vi "Initialize Attributes.vi"(8 "error in (no error)":errorcluster, 10 "Attribute Data":variant, 11 "CS++Fgen in":refnum<class "CS++Fgen.lvclass">) -> (0 "error out":errorcluster, 2 "Found?":bool, 3 "CS++Fgen out":refnum<class "CS++Fgen.lvclass">)   [LabVIEW 2016, in "CS++Fgen.lvlib" / "CS++Fgen.lvclass"]
doc: "Initialize object attribute.\n\nUnique resources should be allocated elsewhere!"
uses:
  CS++Fgen.lvclass
  C:/User/Brand/LVP/CSPP-Dev/Packages/CSPP_Core/Actors/CS++BaseActor/CS++BaseActor.lvclass
  PV-Enum.ctl
  PV-Enum-n.ctl
  CSPP_Core/Classes/CS++ProcessVariables/ProcessVariable/PV.lvclass
  CSPP_Core/Actors/CS++BaseActor/CS++BaseActor.lvclass/CS++BaseActor.ctl
  CSPP_Core/Classes/CS++ProcessVariables/ProcessVariable/PV.lvclass/PV.ctl
  CS++Fgen.lvclass/CS++Fgen.ctl
  CSPP_Core/Classes/CS++ProcessVariables/ProcessVariable/Write PV URL.vi
  CSPP_Core/Classes/CS++ProcessVariables/ProcessVariable/Write Type Descriptor.vi
  <vilib>/Utility/error.llb/Error Cluster From Error Code.vi
  CSPP_Core/Actors/CS++DeviceActor/CS++DeviceActor.lvclass
  CSPP_Core/Classes/CS++BaseClasses/Factory/CS++Factory.lvclass
  CSPP_Core/Actors/CS++BaseActor/CS++BaseActor.lvclass
  CSPP_Core/Libraries/Utilities/CS++Utilities.lvlib
  CSPP_Core/Classes/CS++ProcessVariables/CS++ProcessVariables.lvlib
panel:
  in  "PV-Enum-n":T1
  in  "PV-Enum":T2
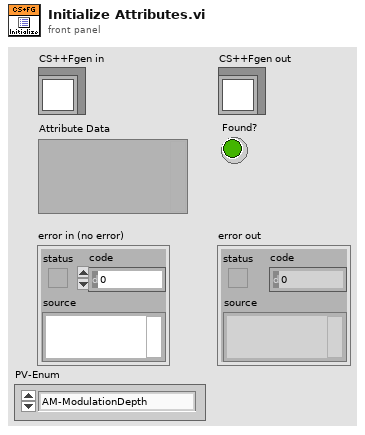
[diagram p1: front panel]
types:
  T1 = typedef "CS++Fgen.lvlib/CS++Fgen.lvclass/PV-Enum-n.ctl" = enum16{"Amplitude", "Arb-Frequency", "DCOffset", "Frequency", "OutputImpedance", "StartPhase", "AdvancedTriggerSlope", "AM-Source", "BurstCount", "FM-Source", "OperationMode", "ResumeTriggerSlope", "StartTriggerSlope", "StopTriggerSlope", "Waveform", "TriggerSource", "AM-Enabled", "ChannelEnabled", "FM-Enabled", "AdvancedTriggerSource", "ResumeTriggerSource", "StartTriggerSource", "StopTriggerSource"}
  T2 = typedef "CS++Fgen.lvlib/CS++Fgen.lvclass/PV-Enum.ctl" = enum16{"AM-ModulationDepth", "AM-ModulationFrequency", "FM-ModulationFrequency", "FP-PeakDeviation", "SampleRate", "TriggerRate", "AM-ModulationWaveform", "FM-ModulationWaveform", "OutputMode", "ReferenceClockSource", "SampleClockSource", "SampleClockOutputEnabled"}
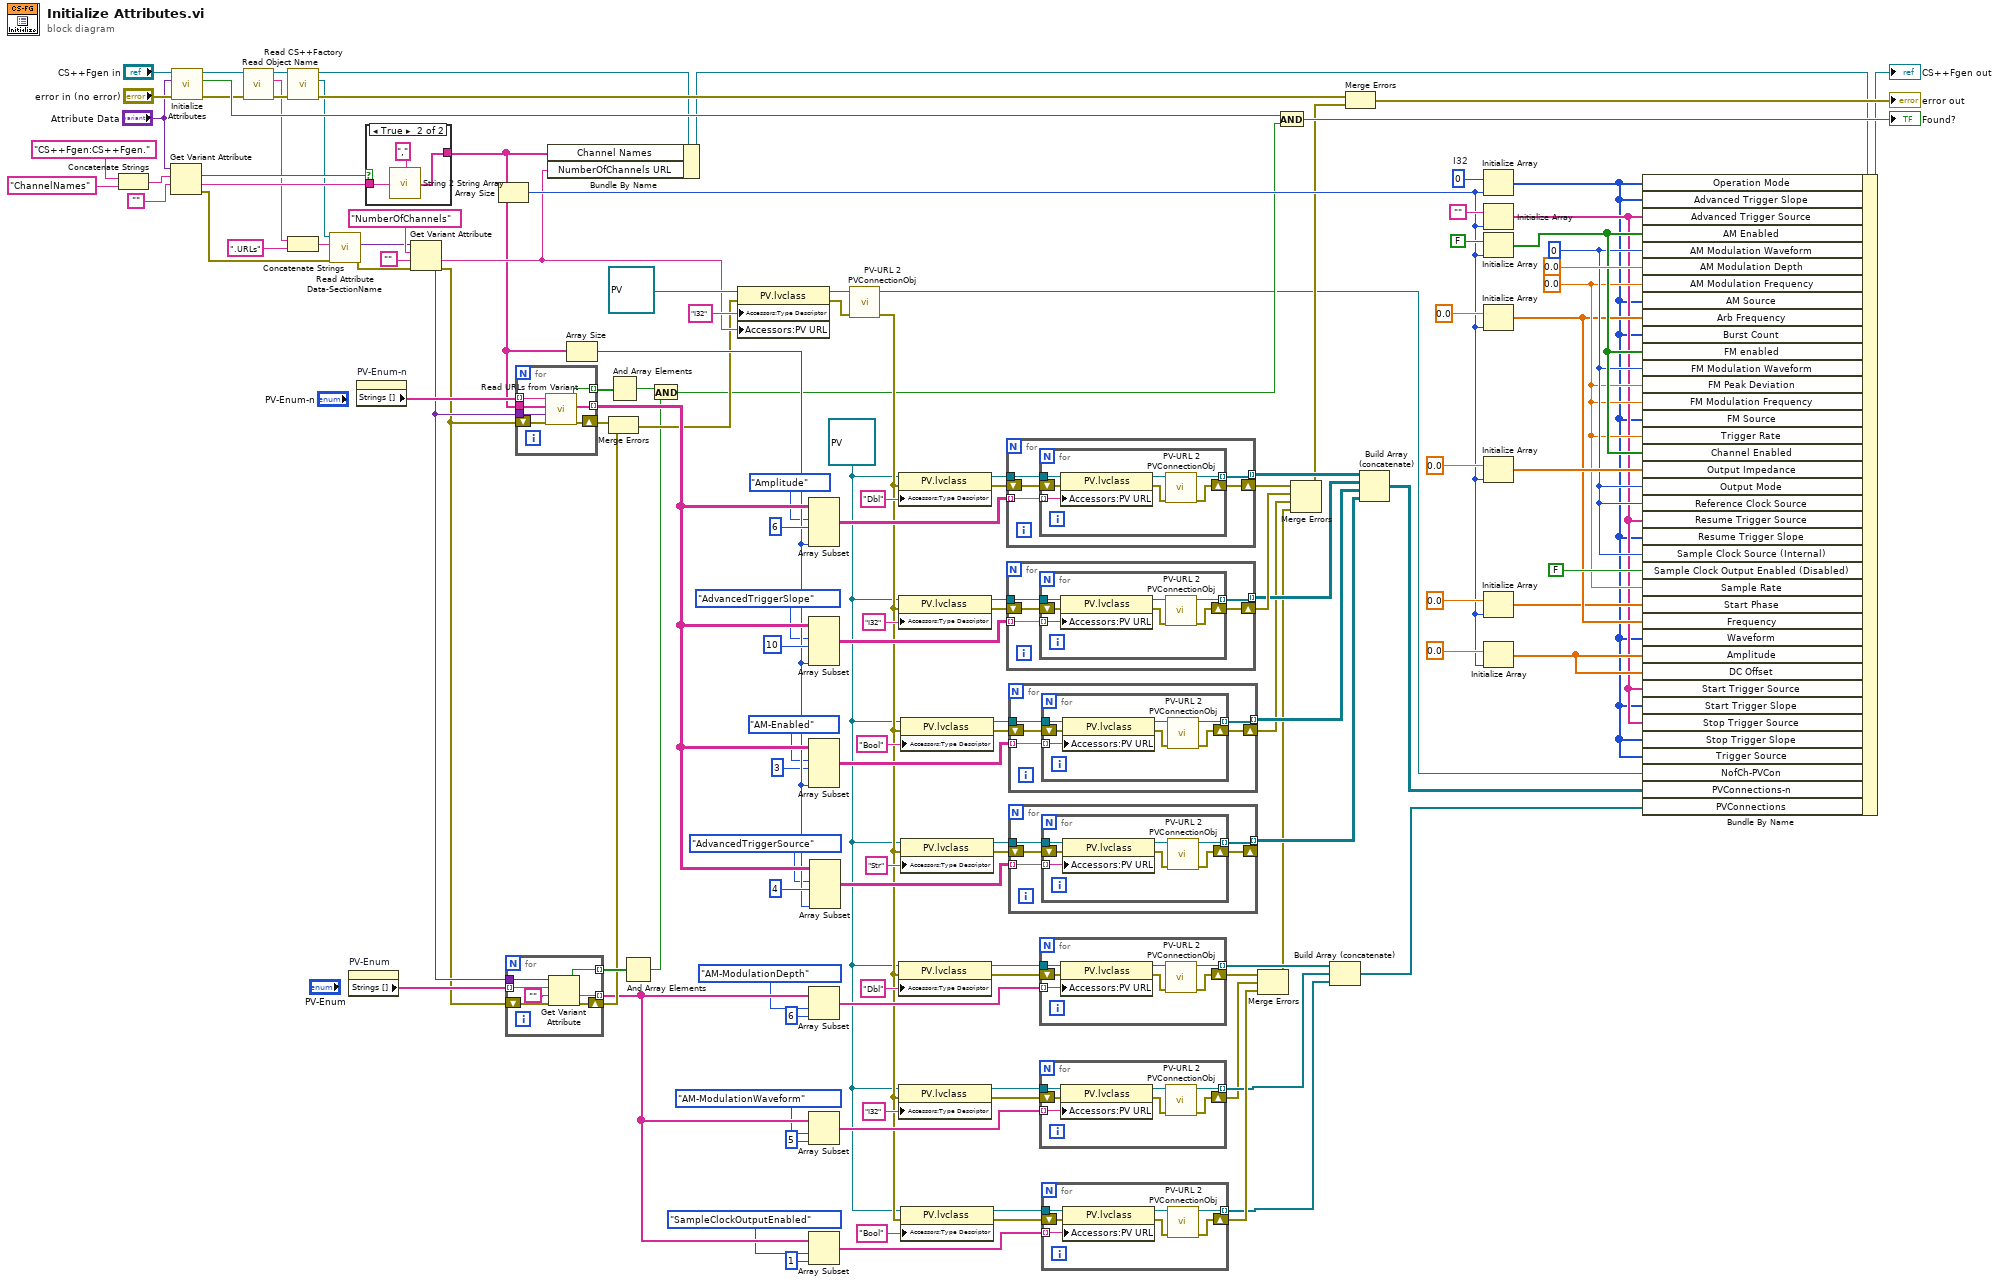
[diagram p0: block diagram]
diagram:
  w23 = refnum<class "PV.lvclass"> refnum ("CS++ProcessVariables.lvlib:PV.lvclass")
  w100 = dbl[unit] 0.0 ("modulation depth (0.00 %)")
  w102 = 0 ("I32")
  w111 = 0  # I32
  n1 = Concatenate Strings("CS++Fgen:CS++Fgen.", "ChannelNames" ("string")) -> (w120:string)
  n2 = Get Variant Attribute(Variant="Attribute Data", name=w120, default value (empty Variant)="") -> (found=w123:bool, value=w122:string, error out=w3:errorcluster)  [unwired: 1 in, 1 out]
  n3 = call-parent "Initialize Attributes.vi"("error in (no error)"="error in (no error)", "Attribute Data"="Attribute Data", "CS++DeviceActor in"="CS++Fgen in") -> ("error out"=w126:errorcluster, "Found?"=w129:bool, "CS++DeviceActor out"=w91:refnum<class "CS++Fgen.lvclass">)  [unwired: 6 in]
  n4 = call "Read Object Name.vi"("error in (no error)"=w126, "CS++BaseActor in"=w91) -> ("error out"=w127:errorcluster, "Object Name"=w12:string, "CS++BaseActor out"=w128:refnum<class "CS++Fgen.lvclass">)  [unwired: 7 in]
  n5 = call "Read CS++Factory.vi"("error in (no error)"=w127, "CS++BaseActor in"=w128) -> ("error out"=w125:errorcluster, "CS++Factory"=w5:refnum<class "CS++Factory.lvclass">, "CS++BaseActor out"=w117:refnum<class "CS++Fgen.lvclass">)  [unwired: 7 in]
  n6 = Concatenate Strings(w12, ".URLs" ("string")) -> (w4:string)
  n7 = call-dynamic "Read Attribute Data-SectionName.vi"("error in (no error)"=w3, "Object Name"=w4, "CS++Factory in"=w5) -> ("error out"=w2:errorcluster, "Attribute Data"=w1:variant)  [unwired: 6 in, 1 out]
  n8 = property on="PV-Enum" class="Enum (strict)"() -> ("Strings []"=w62:string[])  [unwired: 2 in, 2 out]
  n9 = property on="PV-Enum-n" class="Enum (strict)"() -> ("Strings []"=w63:string[])  [unwired: 2 in, 2 out]
  n10 = case shown="True" w123 {
    tunnel: w122 -> [_ w134]
    tunnel: [_ w133] -> w6
    frame False {
    }
    frame True {
      n11 = call "String 2 String Array.vi"("String"=w134, "Delimiter (\",\")"="," ("Delimiter (\",\")")) -> ("Substrings"=w133:string[])
    }
  }
  n12 = Get Variant Attribute(Variant=w1, name="NumberOfChannels" ("string"), default value (empty Variant)="", error in=w2) -> (duplicate Variant=w61:variant, value=w86:string, error out=w60:errorcluster)  [unwired: 1 out]
  n13 = Array Size(array=w6) -> (size(s)=w95:i32)
  n14 = for {
    tunnel: w62 -> [w138] mode=indexing
    tunnel: w61 -> [w139]
    shift-right: [w141] -> w26
    shift-left: w60 -> [w140]
    tunnel: [w137] -> w28 mode=indexing
    tunnel: [w135] -> w25 mode=indexing
    n15 = Get Variant Attribute(Variant=w139, name=w138, default value (empty Variant)="", error in=w140) -> (found=w137:bool, value=w135:string, error out=w141:errorcluster)  [unwired: 1 out]
  }
  n16 = for {
    tunnel: w63 -> [w142] mode=indexing
    tunnel: [w148] -> w85 mode=indexing
    tunnel: w61 -> [w146]
    tunnel: w6 -> [w145]
    tunnel: [w144] -> w51 mode=indexing
    shift-right: [w147] -> w64
    shift-left: w60 -> [w143]
    n17 = call "Read URLs from Variant.vi"("Error In"=w143, "URL Section Data"=w146, "Channel Names"=w145, "URL Prefix"=w142) -> ("Error Out"=w147:errorcluster, "URLs"=w144:string[], "Found?"=w148:bool)  [unwired: 4 in, 1 out]
  }
  n18 = Bundle By Name(cluster=w117, "Channel Names"=w6, "NumberOfChannels URL"=w86) -> (w59:refnum<class "CS++Fgen.lvclass">)
  n19 = Array Size(array=w6) -> (size(s)=w50:i32)
  n20 = Merge Errors(w64, w26) -> (w27:errorcluster)
  n21 = And Array Elements(Boolean array=w85) -> (logical AND=w57:bool)
  n22 = And Array Elements(Boolean array=w28) -> (logical AND=w20:bool)
  n23 = And(x=w57, y=w20) -> (x .and. y?=w21:bool)
  n24 = property class="PV.lvclass"(reference=refnum<class "PV.lvclass"> refnum ("CS++ProcessVariables.lvlib:PV.lvclass"), error in=w27, "Accessors:Type Descriptor"="I32" ("Type Descriptor"), "Accessors:PV URL"=w86) -> (reference out=w87:refnum<class "PV.lvclass">, error out=w88:errorcluster)
  n25 = Array Subset(array=w51, index (row)=PV-Enum-n."Amplitude" ("PV-Enum-n"), length (row)=6 ("length"), length (col)=w50) -> (w84:string[][])  [unwired: 1 in]
  n26 = Array Subset(array=w51, index (row)=PV-Enum-n."AdvancedTriggerSlope" ("PV-Enum-n"), length (row)=10 ("length"), length (col)=w50) -> (w73:string[][])  [unwired: 1 in]
  n27 = Array Subset(array=w51, index (row)=PV-Enum-n."AM-Enabled" ("PV-Enum-n"), length (row)=3 ("length"), length (col)=w50) -> (w72:string[][])  [unwired: 1 in]
  n28 = Array Subset(array=w25, index=PV-Enum."AM-ModulationDepth" ("PV-Enum"), length=6) -> (w29:string[])
  n29 = Array Subset(array=w25, index=PV-Enum."AM-ModulationWaveform" ("PV-Enum"), length=5) -> (w40:string[])
  n30 = Array Subset(array=w25, index=PV-Enum."SampleClockOutputEnabled" ("PV-Enum"), length=1) -> (w41:string[])
  n31 = Array Subset(array=w51, index (row)=PV-Enum-n."AdvancedTriggerSource" ("PV-Enum-n"), length (row)=4 ("length"), length (col)=w50) -> (w52:string[][])  [unwired: 1 in]
  n32 = call "PV-URL 2 PVConnectionObj.vi"("Error In"=w88, "PV"=w87) -> ("Error Out"=w24:errorcluster, "PVConnection"=w19:refnum<class "PVConnection.lvclass">)  [unwired: 7 in, 1 out]
  n33 = property class="PV.lvclass"(reference=w23, error in=w24, "Accessors:Type Descriptor"="Dbl" ("Type Descriptor")) -> (reference out=w82:refnum<class "PV.lvclass">, error out=w81:errorcluster)
  n34 = property class="PV.lvclass"(reference=w23, error in=w24, "Accessors:Type Descriptor"="I32" ("Type Descriptor")) -> (reference out=w77:refnum<class "PV.lvclass">, error out=w78:errorcluster)
  n35 = property class="PV.lvclass"(reference=w23, error in=w24, "Accessors:Type Descriptor"="Dbl" ("Type Descriptor")) -> (reference out=w31:refnum<class "PV.lvclass">, error out=w32:errorcluster)
  n36 = property class="PV.lvclass"(reference=w23, error in=w24, "Accessors:Type Descriptor"="I32" ("Type Descriptor")) -> (reference out=w36:refnum<class "PV.lvclass">, error out=w35:errorcluster)
  n37 = property class="PV.lvclass"(reference=w23, error in=w24, "Accessors:Type Descriptor"="Bool" ("Type Descriptor")) -> (reference out=w70:refnum<class "PV.lvclass">, error out=w69:errorcluster)
  n38 = property class="PV.lvclass"(reference=w23, error in=w24, "Accessors:Type Descriptor"="Str" ("Type Descriptor")) -> (reference out=w54:refnum<class "PV.lvclass">, error out=w55:errorcluster)
  n39 = property class="PV.lvclass"(reference=w23, error in=w24, "Accessors:Type Descriptor"="Bool" ("Type Descriptor")) -> (reference out=w43:refnum<class "PV.lvclass">, error out=w44:errorcluster)
  n40 = for {
    tunnel: w82 -> [w153]
    tunnel: w84 -> [w152] mode=indexing
    tunnel: [w151] -> w79 mode=indexing
    shift-right: [w150] -> w80
    shift-left: w81 -> [w149]
    n41 = for {
      tunnel: w153 -> [w159]
      tunnel: w152 -> [w158] mode=indexing
      tunnel: [w157] -> w151 mode=indexing
      shift-right: [w156] -> w150
      shift-left: w149 -> [w154]
      n42 = property class="PV.lvclass"(reference=w159, error in=w154, "Accessors:PV URL"=w158) -> (reference out=w160:refnum<class "PV.lvclass">, error out=w155:errorcluster)
      n43 = call "PV-URL 2 PVConnectionObj.vi"("Error In"=w155, "PV"=w160) -> ("Error Out"=w156:errorcluster, "PVConnection"=w157:refnum<class "PVConnection.lvclass">)  [unwired: 7 in, 1 out]
    }
  }
  n44 = for {
    tunnel: w77 -> [w165]
    tunnel: w73 -> [w164] mode=indexing
    tunnel: [w163] -> w74 mode=indexing
    shift-right: [w162] -> w75
    shift-left: w78 -> [w161]
    n45 = for {
      tunnel: w165 -> [w171]
      tunnel: w164 -> [w170] mode=indexing
      tunnel: [w169] -> w163 mode=indexing
      shift-right: [w168] -> w162
      shift-left: w161 -> [w166]
      n46 = property class="PV.lvclass"(reference=w171, error in=w166, "Accessors:PV URL"=w170) -> (reference out=w172:refnum<class "PV.lvclass">, error out=w167:errorcluster)
      n47 = call "PV-URL 2 PVConnectionObj.vi"("Error In"=w167, "PV"=w172) -> ("Error Out"=w168:errorcluster, "PVConnection"=w169:refnum<class "PVConnection.lvclass">)  [unwired: 7 in, 1 out]
    }
  }
  n48 = for {
    tunnel: w70 -> [w177]
    tunnel: w72 -> [w176] mode=indexing
    tunnel: [w175] -> w68 mode=indexing
    shift-right: [w174] -> w67
    shift-left: w69 -> [w173]
    n49 = for {
      tunnel: w177 -> [w183]
      tunnel: w176 -> [w182] mode=indexing
      tunnel: [w181] -> w175 mode=indexing
      shift-right: [w180] -> w174
      shift-left: w173 -> [w178]
      n50 = property class="PV.lvclass"(reference=w183, error in=w178, "Accessors:PV URL"=w182) -> (reference out=w184:refnum<class "PV.lvclass">, error out=w179:errorcluster)
      n51 = call "PV-URL 2 PVConnectionObj.vi"("Error In"=w179, "PV"=w184) -> ("Error Out"=w180:errorcluster, "PVConnection"=w181:refnum<class "PVConnection.lvclass">)  [unwired: 7 in, 1 out]
    }
  }
  n52 = for {
    tunnel: w54 -> [w189]
    tunnel: w52 -> [w188] mode=indexing
    tunnel: [w187] -> w22 mode=indexing
    shift-right: [w186] -> _
    shift-left: w55 -> [w185]
    n53 = for {
      tunnel: w189 -> [w195]
      tunnel: w188 -> [w194] mode=indexing
      tunnel: [w193] -> w187 mode=indexing
      shift-right: [w192] -> w186
      shift-left: w185 -> [w190]
      n54 = property class="PV.lvclass"(reference=w195, error in=w190, "Accessors:PV URL"=w194) -> (reference out=w196:refnum<class "PV.lvclass">, error out=w191:errorcluster)
      n55 = call "PV-URL 2 PVConnectionObj.vi"("Error In"=w191, "PV"=w196) -> ("Error Out"=w192:errorcluster, "PVConnection"=w193:refnum<class "PVConnection.lvclass">)  [unwired: 7 in, 1 out]
    }
  }
  n56 = for {
    tunnel: w31 -> [w202]
    tunnel: w29 -> [w201] mode=indexing
    tunnel: [w200] -> w34 mode=indexing
    shift-right: [w199] -> w33
    shift-left: w32 -> [w197]
    n57 = property class="PV.lvclass"(reference=w202, error in=w197, "Accessors:PV URL"=w201) -> (reference out=w203:refnum<class "PV.lvclass">, error out=w198:errorcluster)
    n58 = call "PV-URL 2 PVConnectionObj.vi"("Error In"=w198, "PV"=w203) -> ("Error Out"=w199:errorcluster, "PVConnection"=w200:refnum<class "PVConnection.lvclass">)  [unwired: 7 in, 1 out]
  }
  n59 = for {
    tunnel: w36 -> [w209]
    tunnel: w40 -> [w208] mode=indexing
    tunnel: [w207] -> w39 mode=indexing
    shift-right: [w206] -> w38
    shift-left: w35 -> [w204]
    n60 = property class="PV.lvclass"(reference=w209, error in=w204, "Accessors:PV URL"=w208) -> (reference out=w210:refnum<class "PV.lvclass">, error out=w205:errorcluster)
    n61 = call "PV-URL 2 PVConnectionObj.vi"("Error In"=w205, "PV"=w210) -> ("Error Out"=w206:errorcluster, "PVConnection"=w207:refnum<class "PVConnection.lvclass">)  [unwired: 7 in, 1 out]
  }
  n62 = for {
    tunnel: w43 -> [w216]
    tunnel: w41 -> [w215] mode=indexing
    tunnel: [w214] -> w45 mode=indexing
    shift-right: [w213] -> w46
    shift-left: w44 -> [w211]
    n63 = property class="PV.lvclass"(reference=w216, error in=w211, "Accessors:PV URL"=w215) -> (reference out=w217:refnum<class "PV.lvclass">, error out=w212:errorcluster)
    n64 = call "PV-URL 2 PVConnectionObj.vi"("Error In"=w212, "PV"=w217) -> ("Error Out"=w213:errorcluster, "PVConnection"=w214:refnum<class "PVConnection.lvclass">)  [unwired: 7 in, 1 out]
  }
  n65 = Merge Errors(w33, w38, w46) -> (w16:errorcluster)
  n66 = Compound Arithmetic op=AND(w129, w21) -> (→"Found?":bool)
  n67 = Merge Errors(w80, w75, w67, w16) -> (w58:errorcluster)
  n68 = Build Array (concatenate)(w34, w39, w45) -> (w17:refnum<class "PVConnection.lvclass">[])
  n69 = Merge Errors(w125, w58) -> (→"error out":errorcluster)
  n70 = Build Array (concatenate)(w79, w74, w68, w22) -> (w18:refnum<class "PVConnection.lvclass">[][])
  n71 = Initialize Array(w111, w95) -> (w92:i32[])
  n72 = Initialize Array("" ("output state (Constant Voltage)"), w95) -> (w93:string[])
  n73 = Initialize Array(FALSE, w95) -> (w105:bool[])
  n74 = Initialize Array(dbl[unit] 0.0 ("modulation depth (0.00 %)"), w95) -> (w99:dbl[unit][])
  n75 = Initialize Array(dbl[unit] 0.0 ("modulation depth (0.00 %)"), w95) -> (w103:dbl[unit][])
  n76 = Initialize Array(dbl[unit] 0.0 ("modulation depth (0.00 %)"), w95) -> (w97:dbl[unit][])
  n77 = Initialize Array(dbl[unit] 0.0 ("modulation depth (0.00 %)"), w95) -> (w94:dbl[unit][])
  n78 = Bundle By Name(cluster=w59, "Operation Mode"=w92, "Advanced Trigger Slope"=w92, "Advanced Trigger Source"=w93, "AM Enabled"=w105, "AM Modulation Waveform"=w102, "AM Modulation Depth"=0.0 ("modulation depth (0.00 %)"), "AM Modulation Frequency"=w100, "AM Source"=w92, "Arb Frequency"=w99, "Burst Count"=w92, "FM enabled"=w105, "FM Modulation Waveform"=w102, "FM Peak Deviation"=w100, "FM Modulation Frequency"=w100, "FM Source"=w92, "Trigger Rate"=w100, "Channel Enabled"=w105, "Output Impedance"=w103, "Output Mode"=w102, "Reference Clock Source"=w102, "Resume Trigger Source"=w93, "Resume Trigger Slope"=w92, "Sample Clock Source (Internal)"=w102, "Sample Clock Output Enabled (Disabled)"=FALSE, "Sample Rate"=w100, "Start Phase"=w97, "Frequency"=w99, "Waveform"=w92, "Amplitude"=w94, "DC Offset"=w94, "Start Trigger Source"=w93, "Start Trigger Slope"=w92, "Stop Trigger Source"=w93, "Stop Trigger Slope"=w92, "Trigger Source"=w92, "NofCh-PVCon"=w19, "PVConnections-n"=w18, "PVConnections"=w17) -> (→"CS++Fgen out":refnum<class "CS++Fgen.lvclass">)
